vi "Main.vi"(11 "Module Admin":refnum<class "Delacor_lib_QMH_Module Admin.lvclass">) -> ()   [LabVIEW 2025, in "SafetyLight.lvlib"]
doc: "This template is based off of the Queued Message Handler design pattern and the Queued Message Handler project template that ships with LabVIEW.\n\nThe main difference is that the queue is private to this module and communication between modules is performed via Broadcast and Request events.\n\nRequest events are wrapped in public API methods and are handled in the Event Handling Loop (EHL) of this VI. Any module can register for Broadcast events sent by this module. The EHL generates messages based on user interface actions.\n\nThe Message Handling Loop (MHL) processes messages generated by the EHL, or by other messages. The messages are string values, so new messages can be added easily to the Message Cases case structure in the MHL. Each message cluster can also provide an optional value for Message Data, which is a variant that can be converted to whatever message-specific data is required.\n_____\nBased on DQMH Dev Tools: Project Template 7.1.0.1503."
uses:
  SafetyLight.lvlib
  <vilib>/Delacor/Delacor QMH/Libraries/Module Admin_class/Delacor_lib_QMH_Module Admin.lvclass
  <vilib>/Delacor/Delacor QMH/Libraries/Message Queue_class/Delacor_lib_QMH_Message Queue.lvclass/Delacor_lib_QMH_Message Queue.ctl
  Stop Argument--cluster.ctl
  <vilib>/Delacor/Delacor QMH/Libraries/Module Admin_class/Delacor_lib_QMH_Module Admin.lvclass/Delacor_lib_QMH_Module Admin.ctl
  <vilib>/Utility/miscctls.llb/LVPointTypeDef.ctl
  Test Threshold Argument--cluster.ctl
  <vilib>/Delacor/Delacor QMH/Libraries/Message Queue_class/Delacor_lib_QMH_Enqueue Message (Single).vi
  <vilib>/Delacor/Delacor QMH/Libraries/Module Admin_class/Delacor_lib_QMH_Get External Launch.vi
  <vilib>/Delacor/Delacor QMH/Libraries/Message Queue_class/Delacor_lib_QMH_Message Queue.lvclass
panel:
  out "error out":errorcluster
  out "Status":string
  in  "Simulate MHL Error":bool
  in  "Simulate EHL Error":bool
  # "Other processes communicate with this Module via its Public API (wrappers for its Request Events).\n\nThis Module communicates with other processes via its Broadcast Events.\nAny process that wants to receive these messages can register for this module's Broadcast events."
  # "This template is for the DQMH framework. See the block diagram for more information on how to use this template."
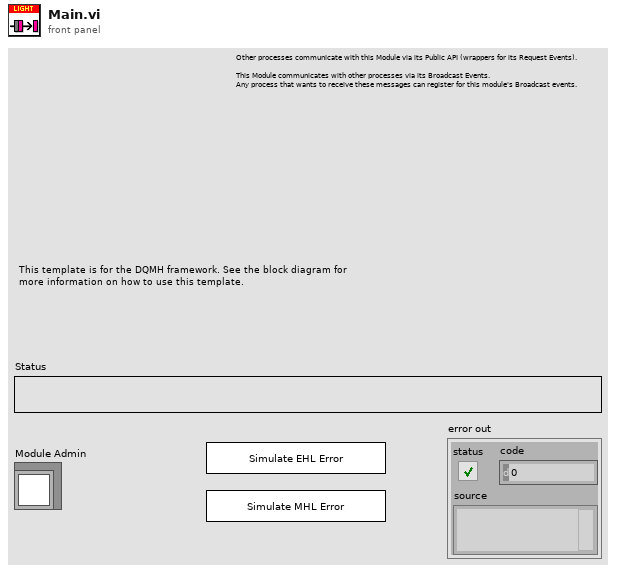
[diagram p1: front panel]
types:
  T1 = typedef "SafetyLight.lvlib/Request Events--cluster.ctl" = cluster{"Stop Module":refnum<user-event>, "Show Panel":refnum<user-event>, "Hide Panel":refnum<user-event>, "Get Module Execution Status":refnum<user-event>, "Show Diagram":refnum<user-event>, "Test Threshold":refnum<user-event>, "TestLight":refnum<user-event>}
  T2 = enum32{"invalid lock state", "Not Locked", "Locked (No Password)", "Password-protected"}
  T3 = typedef "SafetyLight.lvlib/Stop Argument--cluster.ctl" = cluster{"Origin":string, "Exit via Stop Module Req?":bool, "Wait for Module to stop?":bool}
  T4 = typedef "LVPointTypeDef.ctl" = cluster{"Horizontal":i16, "Vertical":i16}
  T5 = enum32{"Invalid", "Standard", "Closed", "Hidden", "Minimized", "Maximized"}
  T6 = typedef "SafetyLight.lvlib/Test Threshold Argument--cluster.ctl" = cluster{"Numeric":dbl}
  T7 = typedef "safety light settings.ctl" = cluster{"Status":string, "Light Status":bool, "Threshold On":dbl, "Threshold Off":dbl, "Siren on time":dbl, "Siren off time":dbl, "Repeats":i32, "repeat interval":dbl}
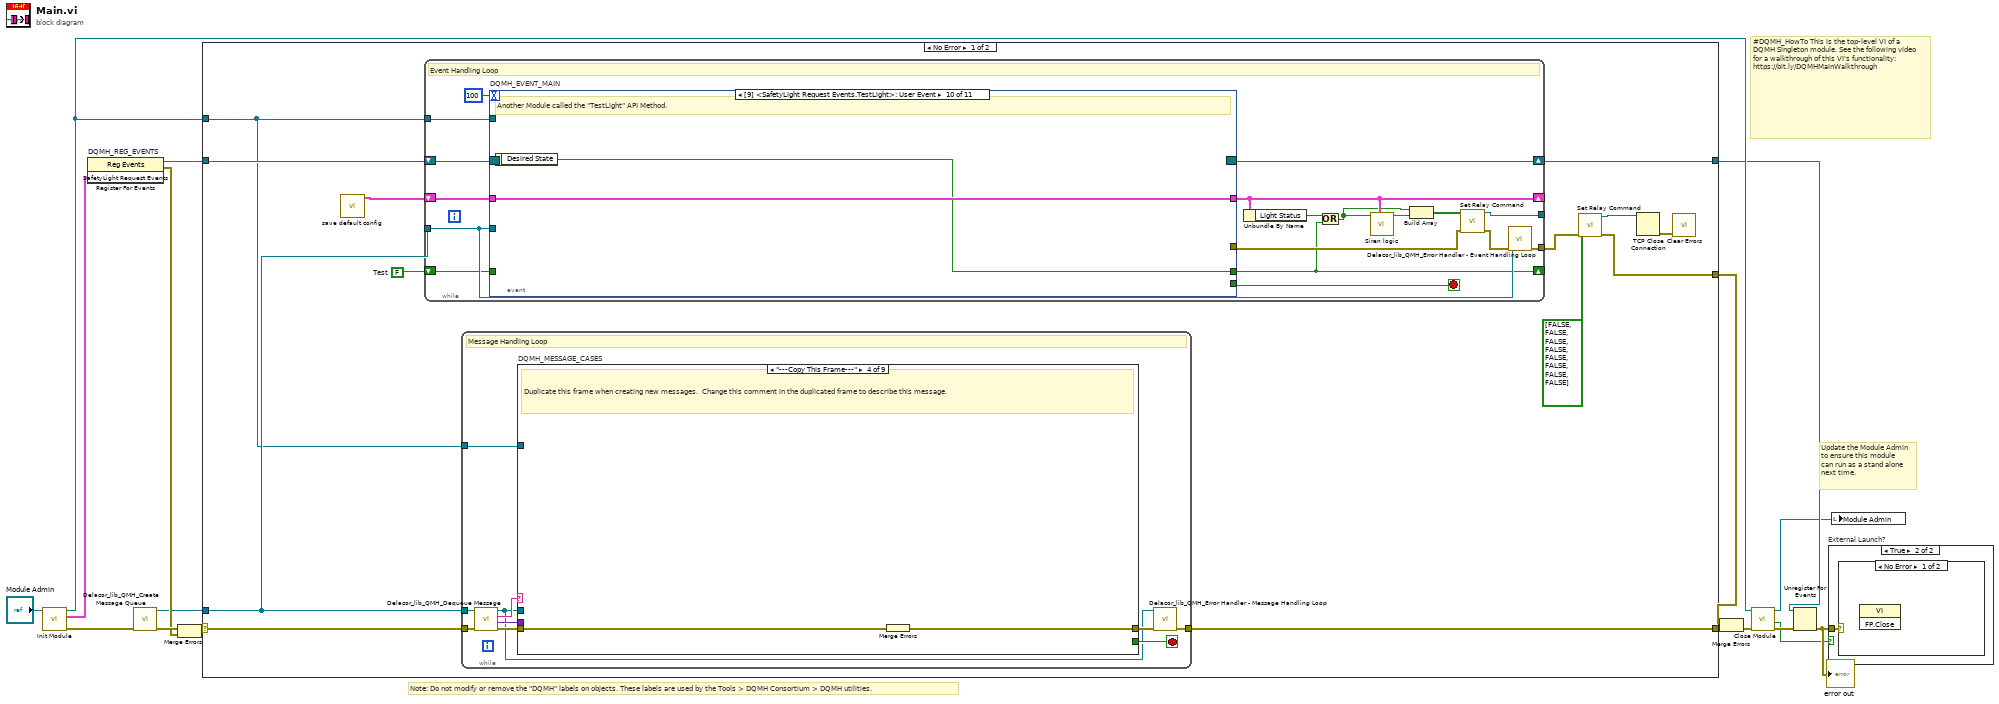
[diagram p0: block diagram]
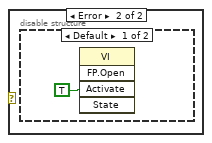
[diagram p3: hidden frame]
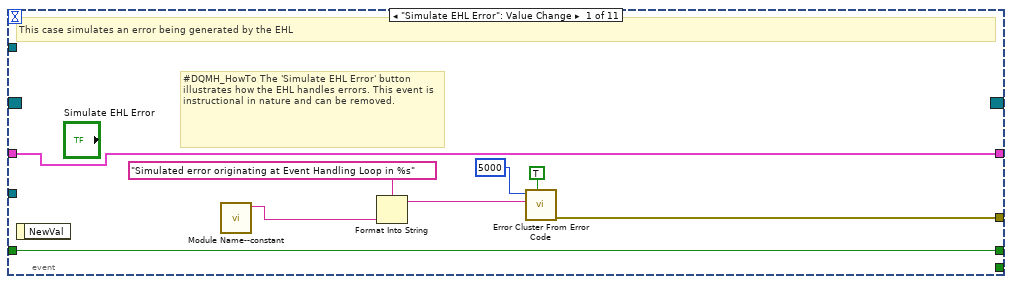
[diagram p5: hidden frame]
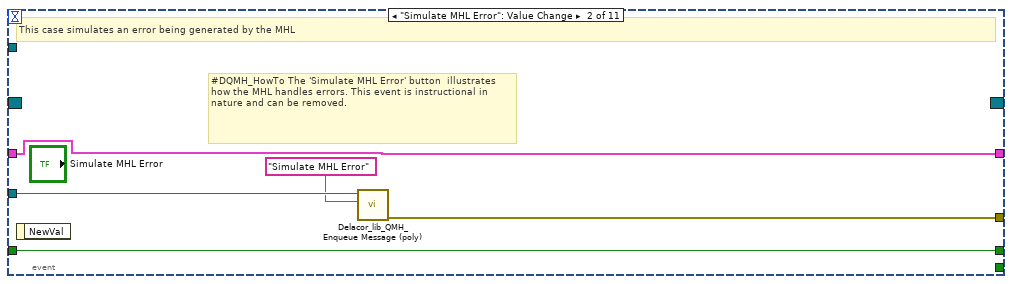
[diagram p6: hidden frame]
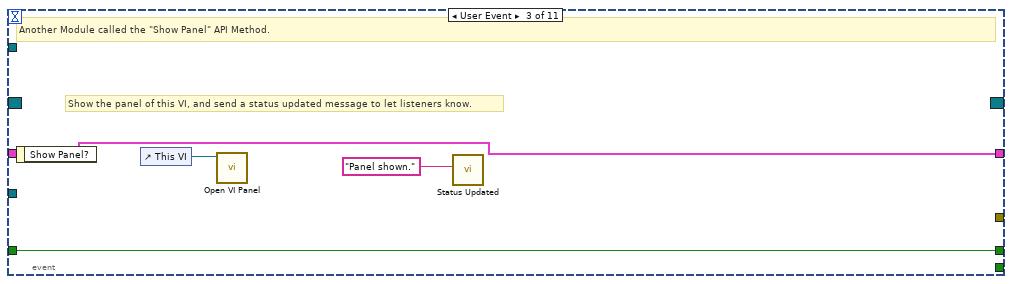
[diagram p7: hidden frame]
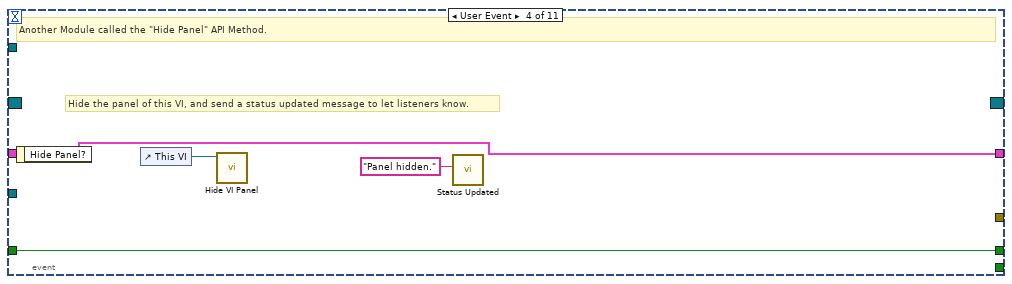
[diagram p8: hidden frame]
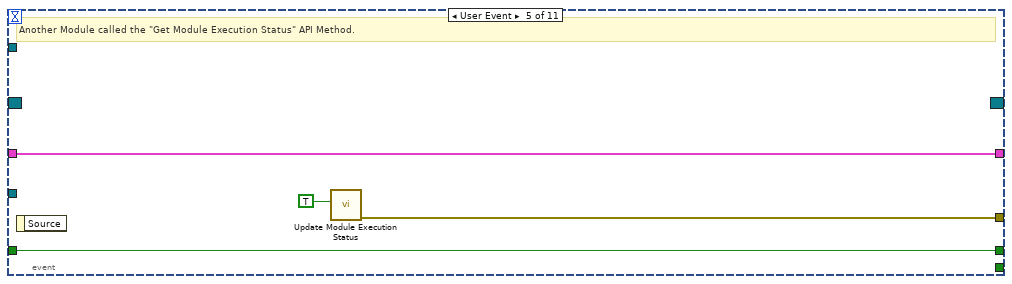
[diagram p9: hidden frame]
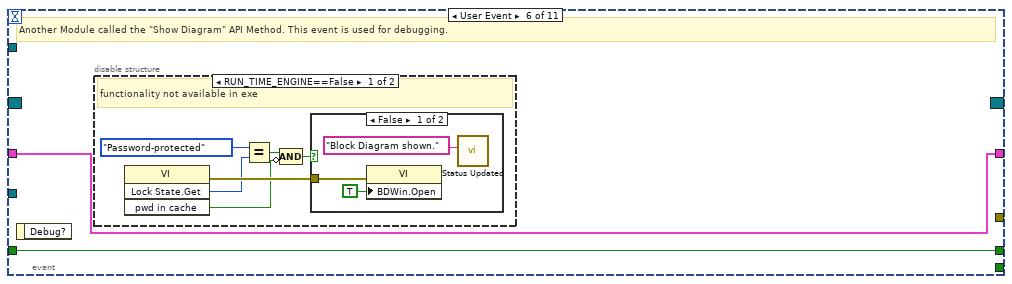
[diagram p10: hidden frame]
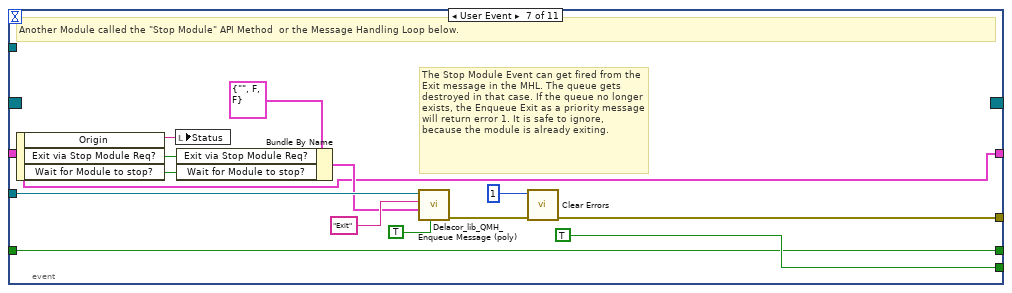
[diagram p13: hidden frame]
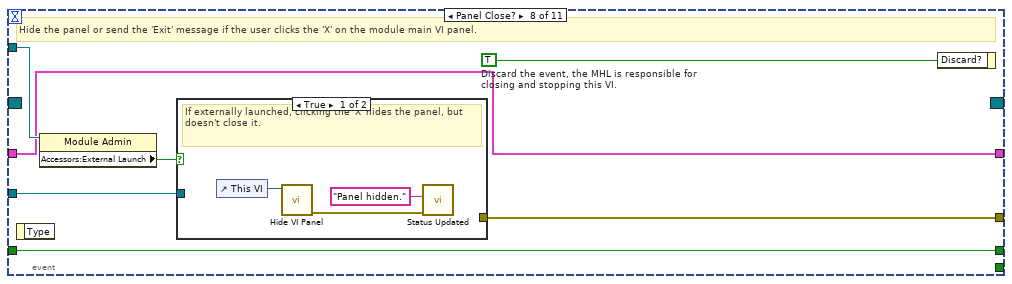
[diagram p14: hidden frame]
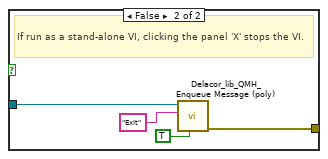
[diagram p15: hidden frame]
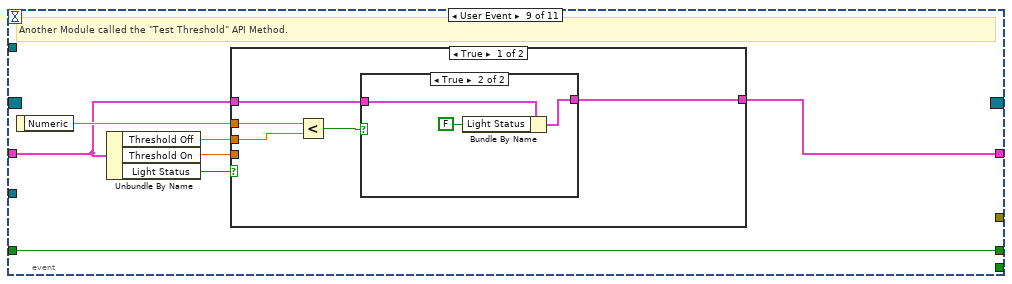
[diagram p16: hidden frame]
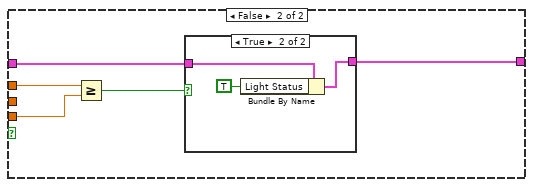
[diagram p18: hidden frame]
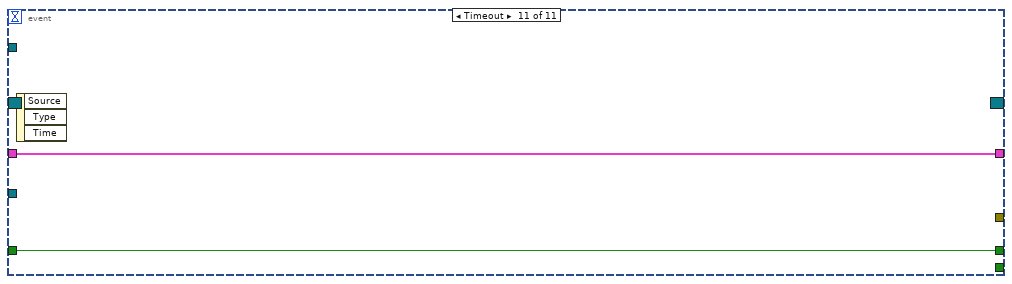
[diagram p20: hidden frame]
diagram:
  # "#DQMH_HowTo This is the top-level VI of a DQMH Singleton module. See the following video for a walkthrough of this VI's functionality: https://bit.ly/DQMHMainWalkthrough"
  # "Note: Do not modify or remove the \"DQMH\" labels on objects. These labels are used by the Tools > DQMH Consortium > DQMH utilities."
  # "Update the Module Admin to ensure this module can run as a stand alone next time."
  n1 = call "Init Module.vi"("Singleton Module Admin in"="Module Admin") -> ("error out"=w16:errorcluster, "SafetyLight Request Events"=w5:T1, "Singleton Module Admin out"=w8:refnum<class "Delacor_lib_QMH_Module Admin.lvclass">)  [unwired: 8 in]
  n2 = register-events "DQMH_REG_EVENTS"(w5) -> (reference out=w6:refnum<event-registration>, error out=w9:errorcluster)  [unwired: 2 in]
  n3 = call <vilib>:"Delacor_lib_QMH_Create Message Queue.vi"("error in"=w16) -> ("error out"=w11:errorcluster, "Message Queue"=w4:refnum<class "Delacor_lib_QMH_Message Queue.lvclass">)  [unwired: 9 in]
  n4 = Merge Errors(w11, w9) -> (w10:errorcluster)
  n5 = case shown="No Error" w10 {
    selector: w10 -> [w29 w233]
    tunnel: [w30 w232] -> w17
    tunnel: [w28 w231] -> w7
    tunnel: w6 -> [w27 w231]
    tunnel: w4 -> [w26 w226]
    tunnel: [w19 _] -> w14
    tunnel: w8 -> [w25 w227]
    frame No Error {
      w18 = FALSE  # Test
      n6 = call "save default config.vi"() -> ("Data out"=w23:T7)  [unwired: 11 in]
      n7 = while {
        tunnel: w26 -> [w43]
        shift-right: [w46] -> w28
        shift-left: w27 -> [w47]
        tunnel: [w48] -> w20
        tunnel: w25 -> [w44]
        shift-right: [w36] -> _
        shift-left: w23 -> [w42]
        tunnel: [w38] -> _
        shift-right: [w32] -> _
        shift-left: w18 -> [w31]
        stop <- w45 stop-if-true
        # "Event Handling Loop"
        n8 = event "DQMH_EVENT_MAIN" shown="[9] <SafetyLight Request Events.TestLight>: User Event" {
          selector: w47 -> [_ _ _ _ _ _ _ _ _ _ _]
          dyn-events: [_ _ _ _ _ _ _ _ _ _ _] -> w46
          timeout: 100 -> [_ _ _ _ _ _ _ _ _ _ _]
          tunnel: [_ _ _ _ _ _ TRUE ("Discard?") _ _ _ _] -> w45
          tunnel: w43 -> [_ w60 _ _ _ _ w94 w103 _ _ _]
          tunnel: [w56 w61 _ _ w73 _ w97 w105 _ _ _] -> w34
          tunnel: w44 -> [_ _ _ _ _ _ _ w102 _ _ _]
          tunnel: w42 -> [w50 w58 w63 w67 w71 w75 w86 w100 w114 w139 w141]
          tunnel: [w50 w58 w63 w67 w71 w75 w86 w100 w115 w139 w141] -> w36
          tunnel: [w49 w57 w62 w66 w70 w74 w85 w99 w113 w138 w140] -> w32
          tunnel: w31 -> [w49 w57 w62 w66 w70 w74 w85 w99 w113 _ w140]
          event "Simulate EHL Error": Value Change {
            # "#DQMH_HowTo The 'Simulate EHL Error' button  illustrates how the EHL handles errors. This event is instructional in nature and can be removed."
            # "This case simulates an error being generated by the EHL"
            n9 = event-data() -> ()  [unwired: 1 in, 1 out]
            n10 = call "Module Name--constant.vi"() -> ("Module Name"=w53:string)  [unwired: 11 in]
            n11 = Format Into String(format string="Simulated error originating at Event Handling Loop in %s", w53) -> (resulting string=w54:string)  [unwired: 2 in, 1 out]
            n12 = call <vilib>:"Error Cluster From Error Code.vi"("show call chain? (False)"=TRUE, "error message (\"\")"=w54, "error code (0)"=5000) -> ("error out"=w56:errorcluster)  [unwired: 6 in]
          }
          event "Simulate MHL Error": Value Change {
            # "#DQMH_HowTo The 'Simulate MHL Error' button  illustrates how the MHL handles errors. This event is instructional in nature and can be removed."
            # "This case simulates an error being generated by the MHL"
            n13 = event-data() -> ()  [unwired: 1 in, 1 out]
            n14 = call-poly <vilib>:"Delacor_lib_QMH_Enqueue Message (poly).vi"("Message"="Simulate MHL Error", "Message Queue in"=w60) -> ("error out"=w61:errorcluster)  [unwired: 8 in, 1 out]
          }
          event User Event {
            # "Show the panel of this VI, and send a status updated message to let listeners know."
            # "Another Module called the \"Show Panel\" API Method."
            n15 = event-data() -> ()  [unwired: 1 in, 1 out]
            n16 = control-ref of="This VI"() -> (w65:refnum<vi>)
            n17 = call "Open VI Panel.vi"("VI"=w65) -> ()  [unwired: 10 in, 1 out]
            n18 = call "Status Updated.vi"("Status"="Panel shown." ("format string")) -> ()  [unwired: 10 in, 1 out]
          }
          event User Event {
            # "Hide the panel of this VI, and send a status updated message to let listeners know."
            # "Another Module called the \"Hide Panel\" API Method."
            n19 = event-data() -> ()  [unwired: 1 in, 1 out]
            n20 = control-ref of="This VI"() -> (w69:refnum<vi>)
            n21 = call "Hide VI Panel.vi"("VI"=w69) -> ()  [unwired: 10 in, 1 out]
            n22 = call "Status Updated.vi"("Status"="Panel hidden." ("format string")) -> ()  [unwired: 10 in, 1 out]
          }
          event User Event {
            # "Another Module called the \"Get Module Execution Status\" API Method."
            n23 = event-data() -> ()  [unwired: 1 in, 1 out]
            n24 = call "Update Module Execution Status.vi"("Running?"=TRUE) -> ("error out"=w73:errorcluster)  [unwired: 10 in]
          }
          event User Event {
            # "Another Module called the \"Show Diagram\" API Method. This event is used for debugging."
            n25 = event-data() -> ()  [unwired: 1 in, 1 out]
            n26 = disable-structure shown="RUN_TIME_ENGINE==False" {
              frame condition #0 (active) {
                # "functionality not available in exe"
                n27 = invoke on="Invoke Node" class="VI" method="Lock State.Get"() -> (error out=w81:errorcluster, "Get Lock State"=w80:T2, "pwd in cache"=w77:bool)  [unwired: 4 in, 1 out]
                n28 = Equal?(x=T2."Password-protected", y=w80) -> (x = y?=w78:bool)
                n29 = Compound Arithmetic op=AND(w78, invert w77) -> (w76:bool)
                n30 = case shown="False" w76 {
                  tunnel: w81 -> [w84 _]
                  frame False {
                    n31 = property on="Property Node" class="VI"(error in=w84, "BDWin.Open"=TRUE ("Block Diagram Window:Open")) -> ()  [unwired: 1 in, 2 out]
                    n32 = call "Status Updated.vi"("Status"="Block Diagram shown." ("format string")) -> ()  [unwired: 10 in, 1 out]
                  }
                  frame True {
                    # "Password-protected VI, and the password is not in the cache. Do not show the diagram."
                  }
                }
              }
              frame condition #1 {
              }
            }
          }
          event User Event {
            # "The Stop Module Event can get fired from the Exit message in the MHL. The queue gets destroyed in that case. If the queue no longer exists, the Enqueue Exit as a priority message will return error 1. It is safe to ignore, because the module is already exiting."
            # "Another Module called the \"Stop Module\" API Method  or the Message Handling Loop below."
            n33 = event-data() -> ("Origin"=w93:string, "Exit via Stop Module Req?"=w89:bool, "Wait for Module to stop?"=w88:bool)  [unwired: 1 in]
            n34 = local write "Status"(w93) -> ()
            n35 = Bundle By Name(cluster=T3 {"Origin"="", "Exit via Stop Module Req?"=FALSE, "Wait for Module to stop?"=FALSE} ("Stop Argument"), "Exit via Stop Module Req?"=w89, "Wait for Module to stop?"=w88) -> (w87:T3)
            n36 = call-poly <vilib>:"Delacor_lib_QMH_Enqueue Message (poly).vi"("Priority Message? (F)"=TRUE, "Message Data"=w87, "Message"="Exit", "Message Queue in"=w94) -> ("error out"=w98:errorcluster)  [unwired: 6 in, 1 out]
            n37 = call <vilib>:"Clear Errors.vi"("error in (no error)"=w98, "specific error code to clear (0: all)"=1) -> ("error out"=w97:errorcluster)  [unwired: 4 in, 1 out]
          }
          event Panel Close? {
            w104 = TRUE  # Discard the event, the MHL is responsible for closing and stopping this VI.
            # "Hide the panel or send the 'Exit' message if the user clicks the 'X' on the module main VI panel."
            n38 = event-data() -> ()  [unwired: 1 in, 1 out]
            n39 = property on="Property Node" class="Module Admin"(reference=w102) -> ("Accessors:External Launch"=w101:bool)  [unwired: 1 in, 2 out]
            n40 = case shown="True" w101 {
              tunnel: w103 -> [_ w111]
              tunnel: [_ w112] -> w105
              frame True {
                # "If externally launched, clicking the 'X' hides the panel, but doesn't close it."
                n41 = control-ref of="This VI"() -> (w108:refnum<vi>)
                n42 = call "Hide VI Panel.vi"("VI"=w108) -> ("error out"=w106:errorcluster)  [unwired: 10 in]
                n43 = call "Status Updated.vi"("error in"=w106, "Status"="Panel hidden." ("format string")) -> ()  [unwired: 9 in, 1 out]
              }
              frame False {
                # "If run as a stand-alone VI, clicking the panel 'X' stops the VI."
                n44 = call-poly <vilib>:"Delacor_lib_QMH_Enqueue Message (poly).vi"("Priority Message? (F)"=TRUE, "Message"="Exit", "Message Queue in"=w111) -> ("error out"=w112:errorcluster)  [unwired: 7 in, 1 out]
              }
            }
            n45 = event-data ("Event Filter Node")("Discard?"=w104) -> ()  [unwired: 1 in, 1 out]
          }
          event User Event {
            # "Another Module called the \"Test Threshold\" API Method."
            n46 = event-data() -> ("Numeric"=w118:dbl)  [unwired: 1 in]
            n47 = Unbundle By Name(w114) -> ("Threshold Off"=w117:dbl, "Threshold On"=w116:dbl, "Light Status"=w119:bool)
            n48 = case shown="True" w119 {
              tunnel: w118 -> [w124 w133]
              tunnel: w117 -> [w123 _]
              tunnel: w116 -> [_ w129]
              tunnel: w114 -> [w122 w132]
              tunnel: [w120 w130] -> w115
              frame True {
                n49 = Less?(x=w124, y=w123) -> (x < y?=w121:bool)
                n50 = case shown="True" w121 {
                  tunnel: w122 -> [w125 w128]
                  tunnel: [w125 w126] -> w120
                  frame False {
                  }
                  frame True {
                    n51 = Bundle By Name(cluster=w128, "Light Status"=FALSE) -> (w126:T7)
                  }
                }
              }
              frame False {
                n52 = Greater Or Equal?(x=w133, y=w129) -> (x >= y?=w131:bool)
                n53 = case shown="True" w131 {
                  tunnel: w132 -> [w134 w137]
                  tunnel: [w134 w135] -> w130
                  frame False {
                  }
                  frame True {
                    n54 = Bundle By Name(cluster=w137, "Light Status"=TRUE) -> (w135:T7)
                  }
                }
              }
            }
          }
          event User Event {
            # "Another Module called the \"TestLight\" API Method."
            n55 = event-data() -> ("Desired State"=w138:bool)  [unwired: 1 in]
          }
          event Timeout {
            n56 = event-data() -> ()  [unwired: 1 in, 3 out]
          }
        }
        n57 = Unbundle By Name(w36) -> ("Light Status"=w40:bool)
        n58 = Or(x=w40, y=w32) -> (x .or. y?=w33:bool)
        n59 = call "Siren logic.vi"("Data out"=w36, "Strobe Light State"=w33) -> ("Siren State Out"=w41:bool)  [unwired: 9 in]
        n60 = Build Array(w33, w41) -> (w39:bool[])
        n61 = call "Set Relay Command.vi"("error in"=w34, "Desired Relay State"=w39) -> ("error out"=w35:errorcluster, "connection ID"=w38:refnum<k5>)  [unwired: 8 in]
        n62 = call-dynamic "Delacor_lib_QMH_Error Handler - Event Handling Loop.vi"("error in"=w35, "Message Queue in"=w43) -> ("dup error in"=w48:errorcluster)  [unwired: 8 in, 1 out]
      }
      n63 = while {
        tunnel: w26 -> [w142]
        tunnel: w29 -> [w151]
        tunnel: [w145] -> w30
        tunnel: w25 -> [w146]
        stop <- w149 stop-if-true
        # "Message Handling Loop"
        n64 = call-dynamic "Delacor_lib_QMH_Dequeue Message.vi"("error in"=w151, "Message Queue in"=w142) -> ("error out"=w150:errorcluster, "Message Data"=w147:variant, "Message"=w148:string, "Message Queue out"=w143:refnum<class "Delacor_lib_QMH_Message Queue.lvclass">)  [unwired: 6 in]
        n65 = case "DQMH_MESSAGE_CASES" shown="\"---Copy This Frame---\"" w148 {
          selector: w148 -> [_ _ _ _ _ _ _ _ w222]
          tunnel: w143 -> [_ _ _ _ _ _ w190 w210 _]
          tunnel: w150 -> [w167 w170 w175 w177 w178 w186 w196 w216 w224]
          tunnel: [w165 w170 w174 w176 w178 w185 w192 w211 w225] -> w144
          tunnel: [_ _ _ _ _ _ _ w209 _] -> w149
          tunnel: w147 -> [_ _ w173 _ _ _ w191 w208 _]
          tunnel: w146 -> [w157 _ _ _ _ _ w189 w203 _]
          frame "Initialize" {
            # "Initialize - Any operation that needs to be done before the module can receive messages. Synchronize Caller Events.vi will inform Start Module.vi that the module has launched and is ready to receive messages. Module Did Init.vi will broadcast that the module initialized."
            n66 = call "Synchronize Caller Events.vi"("error in"=w167, "Singleton Module Admin in"=w157) -> ("error out"=w166:errorcluster, "Singleton Module Admin out"=w154:refnum<class "Delacor_lib_QMH_Module Admin.lvclass">)  [unwired: 8 in]
            n67 = property on="Property Node" class="Module Admin"(reference=w154) -> ("Accessors:External Launch"=w161:bool)  [unwired: 1 in, 2 out]
            n68 = Select(t=T5."Hidden" ("State"), s=w161, f=T5."Standard" ("State")) -> (s? t:f=w158:T5)
            n69 = call "Module Name--constant.vi"() -> ("Module Name"=w164:string)  [unwired: 11 in]
            n70 = property on="Property Node" class="VI"("Front Panel.Title"=w164) -> (reference out=w163:refnum<vi>, error out=w169:errorcluster)  [unwired: 2 in]
            n71 = invoke on="Invoke Node" class="VI" method="FP.Open"(reference=w163, error in=w169, "State"=w158) -> (reference out=w162:refnum<vi>, error out=w168:errorcluster)  [unwired: 2 in, 3 out]
            n72 = invoke on="Invoke Node" class="VI" method="FP.Center"(reference=w162, error in=w168) -> ()  [unwired: 1 in, 3 out]
            n73 = property on="Pane" class="Pane"("Origin"=T4 {"Horizontal"=0, "Vertical"=0}) -> ()  [unwired: 2 in, 2 out]
            n74 = call "Module Name--constant.vi"() -> ("Module Name"=w155:string)  [unwired: 11 in]
            n75 = call "Module Did Init.vi"("error in"=w166, "Initialized?"=TRUE, "Origin"=w155) -> ("error out"=w165:errorcluster)  [unwired: 8 in]
            "Status" <- "Initial Message" ("Initial Message")
          }
          frame "---Module Specific---" {
            # "Separator -- The following cases handle messages specific to this Module."
          }
          frame "Test Threshold" {
            n76 = Variant To Data(error in=w175, type=T6 {"Numeric"=0.0} ("Test Threshold Argument"), Variant=w173) -> (data=w171:T6, error out=w174:errorcluster)
            n77 = Unbundle By Name(w171) -> ()  [unwired: 1 out]
          }
          frame "---Copy This Frame---" {
            # "Duplicate this frame when creating new messages.  Change this comment in the duplicated frame to describe this message."
            n78 = Merge Errors(w177) -> (w176:errorcluster)
          }
          frame "---Exit and Error Handling---" {
            # "Separator - The following cases handle errors and exit messages."
          }
          frame "Simulate MHL Error" {
            # "#DQMH_HowTo The 'Simulate MHL Error' button  illustrates how the MHL handles errors. This event is instructional in nature and can be removed."
            # "Simulate an error occurring at the MHL"
            n79 = call "Module Name--constant.vi"() -> ("Module Name"=w180:string)  [unwired: 11 in]
            n80 = Format Into String(format string="Simulated error originating at Message Handling Loop in %s", w180) -> (resulting string=w181:string)  [unwired: 2 in, 1 out]
            n81 = call <vilib>:"Error Cluster From Error Code.vi"("show call chain? (False)"=TRUE, "error message (\"\")"=w181, "error code (0)"=5001) -> ("error out"=w184:errorcluster)  [unwired: 6 in]
            n82 = Merge Errors(w186, w184) -> (w185:errorcluster)
          }
          frame "Error" {
            # "#DQMH_CodeRecommended - If the module is running in standalone mode (External Launch = FALSE), this code will pop up an error dialog and call the 'Exit' message if an error occurs. Add more fine-grained error management here."
            # "Error - Check the error message data and respond accordingly. This message is sent by the \"Error Handler\" VIs at the end of each loop in this application."
            n83 = property on="Property Node" class="Module Admin"(reference=w189) -> ("Accessors:External Launch"=w188:bool)  [unwired: 1 in, 2 out]
            n84 = Variant To Data(error in=w196, type=errorcluster {"status"=FALSE, "code"=0, "source"=""} ("error constant"), Variant=w191) -> (data=w187:errorcluster, error out=w194:errorcluster)
            n85 = local write "error out"(w187) -> ()
            n86 = call "Error Reported.vi"("Error"=w187) -> ()  [unwired: 10 in, 1 out]
            n87 = case shown="False" w188 {
              tunnel: [w201 _] -> w193
              tunnel: w190 -> [w199 _]
              tunnel: w187 -> [w200 _]
              frame False {
                n88 = disable-structure shown="Default" {
                  disable-tunnel: w200 -> [w202 _]
                  frame condition #0 (active) {
                    # "If the module is running standalone, then pop up an error dialog and call the \"Exit\" message."
                    n89 = call <vilib>:"Simple Error Handler.vi"("error in (no error)"=w202) -> ()  [unwired: 4 in, 5 out]
                  }
                  frame condition #1 {
                    # "To prevent the Simple Error Handler VI from being loaded (e.g. when deploying to a Real-Time target), add the Conditional Disable Symbol \"DQMH_Disable_SEH\" to your project and set it to TRUE."
                  }
                }
                n90 = call-poly <vilib>:"Delacor_lib_QMH_Enqueue Message (poly).vi"("Priority Message? (F)"=TRUE, "Message"="Exit", "Message Queue in"=w199) -> ("error out"=w201:errorcluster)  [unwired: 7 in, 1 out]
              }
              frame True {
                # "If the module was launched externally, calling the Error Reported broadcast VI is the only action performed by the \"Error\" message. The module's caller can then process the error appropriately."
              }
            }
            n91 = Merge Errors(w194, w193) -> (w192:errorcluster)
          }
          frame "Exit" {
            w207 = 91  # 91: not all Exit messages will have an argument
            w209 = TRUE  # Stop the VI
            # "Release the message queue reference"
            # "#DQMH_CodeNeeded - Add any required cleanup code here."
            # "Exit - Exit the application."
            n92 = Variant To Data(error in=w216, type=T3 {"Origin"="", "Exit via Stop Module Req?"=FALSE, "Wait for Module to stop?"=FALSE} ("Stop Argument"), Variant=w208) -> (data=w205:T3, error out=w213:errorcluster)
            n93 = call <vilib>:"Clear Errors.vi"("error in (no error)"=w213, "specific error code to clear (0: all)"=w207) -> ("error out"=w215:errorcluster)  [unwired: 4 in, 1 out]
            n94 = control-ref of="This VI"() -> (w204:refnum<vi>)
            n95 = call-dynamic "Delacor_lib_QMH_Release Message Queue.vi"("error in"=w215, "Message Queue"=w210) -> ("error out"=w214:errorcluster)  [unwired: 9 in]
            n96 = call "Handle Exit.vi"("Stop Argument"=w205, "Admin in"=w203, "VI reference"=w204) -> ("error out"=w212:errorcluster)  [unwired: 7 in, 1 out]
            n97 = Merge Errors(w214, w212) -> (w211:errorcluster)
            n98 = call "Error Reported.vi"("Error"=w211) -> ()  [unwired: 10 in, 1 out]
          }
          frame Default {
            # "'Default' case only runs if there is a message that isn't defined in any of the other cases.  Output a programming error."
            n99 = call "Module Name--constant.vi"() -> ("Module Name"=w221:string)  [unwired: 11 in]
            n100 = Format Into String(format string="The invalid message string \"%s\" was received in the Message Handling Loop for module \"%s\".", w222, w221) -> (resulting string=w217:string)  [unwired: 2 in, 1 out]
            n101 = call <vilib>:"Error Cluster From Error Code.vi"("show call chain? (False)"=TRUE, "error message (\"\")"=w217, "error code (0)"=1) -> ("error out"=w223:errorcluster)  [unwired: 6 in]
            n102 = Merge Errors(w224, w223) -> (w225:errorcluster)
          }
        }
        n103 = call-dynamic "Delacor_lib_QMH_Error Handler - Message Handling Loop.vi"("error in"=w144, "Message Queue in"=w143) -> ("dup error in"=w145:errorcluster)  [unwired: 8 in, 1 out]
      }
      n104 = call "Set Relay Command.vi"("error in"=w20, "Desired Relay State"=bool[] [FALSE, FALSE, FALSE, FALSE, FALSE, FALSE, FALSE, FALSE]) -> ("error out"=w19:errorcluster, "connection ID"=w22:refnum<k5>)  [unwired: 8 in]
      n105 = TCP Close Connection(connection ID=w22) -> (error out=w24:errorcluster)  [unwired: 2 in, 1 out]
      n106 = call <vilib>:"Clear Errors.vi"("error in (no error)"=w24) -> ()  [unwired: 5 in, 2 out]
    }
    frame Error {
      # "Synchronize Caller Events.vi will inform Start Module.vi that the module has launched and will let the code calling Start Module.vi register for broadcasts and would permit the caller receive the broadcast that an error occurred at launch time."
      n107 = call-dynamic "Delacor_lib_QMH_Release Message Queue.vi"("error in"=w233, "Message Queue"=w226) -> ("error out"=w232:errorcluster)  [unwired: 9 in]
      n108 = call "Synchronize Caller Events.vi"("Singleton Module Admin in"=w227) -> ("error out"=w234:errorcluster)  [unwired: 9 in, 1 out]
      n109 = call "Module Name--constant.vi"() -> ("Module Name"=w230:string)  [unwired: 11 in]
      n110 = Format Into String(format string="An error occurred during initialization. %s is no longer running.", w230) -> (resulting string=w228:string)  [unwired: 2 in, 1 out]
      n111 = Merge Errors(w232, w234) -> (w235:errorcluster)
      n112 = call "Error Reported.vi"("Additional Information"=w228, "Error"=w235) -> ()  [unwired: 9 in, 1 out]
    }
  }
  n113 = Merge Errors(w14, w17) -> (w13:errorcluster)
  n114 = call "Close Module.vi"("error in"=w13, "Module Admin in"=w8) -> ("error out"=w15:errorcluster, "External Launch"=w1:bool, "Module Admin out"=w2:refnum<class "Delacor_lib_QMH_Module Admin.lvclass">)  [unwired: 7 in]
  n115 = Unregister For Events(event registration refnum=w7, error in=w15) -> (error out=w12:errorcluster)
  "error out" <- w12
  n116 = case "External Launch?" shown="True" w1 {
    tunnel: w12 -> [_ w236]
    frame False {
    }
    frame True {
      n117 = case shown="No Error" w236 {
        frame No Error {
          n118 = invoke on="Invoke Node" class="VI" method="FP.Close"() -> ()  [unwired: 3 in, 3 out]
        }
        frame Error {
          n119 = disable-structure shown="Default" {
            frame condition #0 (active) {
              n120 = invoke class="VI" method="FP.Open"("Activate"=TRUE ("Activate?")) -> ()  [unwired: 4 in, 5 out]
            }
            frame condition #1 {
              # "Don't show panel on error if running inside a built EXE."
            }
          }
        }
      }
    }
  }
  n121 = local write "Module Admin"(w2) -> ()
